vi "getBounds.vi"(0 "reference":refnum<class "StateDiagramGraph.lvclass">, 1 "graphics":refnum<class "Graphics.lvclass">, 5 "error in (no error)":errorcluster) -> (14 "reference out":refnum<class "StateDiagramGraph.lvclass">, 15 "bounds":T1 {"height" format="%.2f"; "width" format="%.2f"; "y" format="%.2f"; "x" format="%.2f"}, 19 "error out":errorcluster)   [LabVIEW 2014, in "StateDiagramGraph.lvclass"]
doc: "getBounds"
uses:
  <resource>/Framework/Providers/Open_GDS/UML/StateDiagramGraph_class/StateDiagramGraph.lvclass
  <resource>/Framework/Providers/Open_GDS/UML/Graphics_class/Graphics.lvclass
  <resource>/Framework/Providers/Open_GDS/UML/General/Rectangle/Rectangle Rectangle2D.ctl
  <resource>/Framework/Providers/Open_GDS/UML/StateDiagramGraph_class/private/ViPathShowOption.ctl
  <resource>/Framework/Providers/Open_GDS/UML/Graph_class/Graph.lvclass
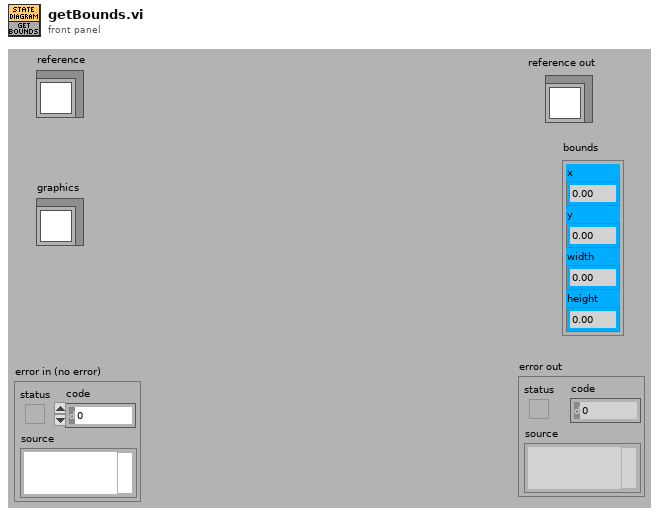
[diagram p1: front panel]
types:
  T1 = typedef "Rectangle Rectangle2D.ctl" = cluster{"x":dbl, "y":dbl, "width":dbl, "height":dbl}
  T2 = typedef "StateDiagramGraph.lvclass/ViPathShowOption.ctl" = enum16{"Don't Show", "Show Relative Path", "Show Absolute Path"}
  T3 = typedef "StateDiagramGraph.lvclass/ObjectAttributes.ctl" = cluster{"StateDiagramData":T4}
  T4 = typedef "StateDiagramGraph.lvclass/StateDiagramData.ctl" = cluster{"VI-Path":path, "ShowOption":T2}
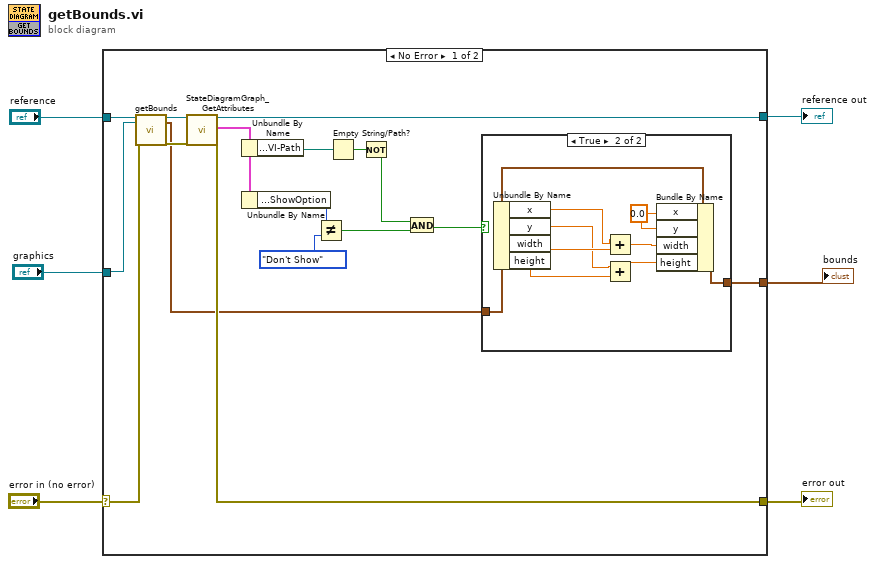
[diagram p0: block diagram]
diagram:
  n1 = case shown="No Error" "error in (no error)" {
    selector: "error in (no error)" -> [w10 w34]
    tunnel: "reference" -> [w13 w35]
    tunnel: [w22 w34] -> w4
    tunnel: [w23 w35] -> w3
    tunnel: "graphics" -> [w9 _]
    tunnel: [w21 _] -> w1
    frame No Error {
      n2 = call-parent "getBounds.vi"("reference"=w13, "graphics"=w9, "error in (no error)"=w10) -> ("reference out"=w12:refnum<class "StateDiagramGraph.lvclass">, "bounds"=w8:T1, "error out"=w11:errorcluster)  [unwired: 14 in]
      n3 = call <resource>:"StateDiagramGraph_GetAttributes.vi"("reference in"=w12, "error in (no error)"=w11) -> ("reference out"=w23:refnum<class "StateDiagramGraph.lvclass">, "Data"=w7:T3, "error out"=w22:errorcluster)  [unwired: 1 in, 14 out]
      n4 = Unbundle By Name(w7) -> ("StateDiagramData.VI-Path"=w17:path)
      n5 = Unbundle By Name(w7) -> ("StateDiagramData.ShowOption"=w20:T2)
      n6 = Not Equal?(x=w20, y=ViPathShowOption."Don't Show") -> (x != y?=w18:bool)
      n7 = Empty String/Path?(string/path=w17) -> (empty?=w16:bool)
      n8 = Not(x=w16) -> (.not. x?=w15:bool)
      n9 = And(x=w15, y=w18) -> (x .and. y?=w14:bool)
      n10 = case shown="True" w14 {
        tunnel: [w24 w33] -> w21
        tunnel: w8 -> [w24 w29]
        frame False {
        }
        frame True {
          w32 = 0.0 ("x")
          n11 = Unbundle By Name(w29) -> ("x"=w28:dbl, "y"=w26:dbl, "width"=w27:dbl, "height"=w25:dbl)
          n12 = Add(x=w28, y=w27) -> (x+y=w31:dbl)
          n13 = Add(x=w26, y=w25) -> (x+y=w30:dbl)
          n14 = Bundle By Name(cluster=w29, "x"=w32, "y"=w32, "width"=w31, "height"=w30) -> (w33:T1)
        }
      }
    }
    frame Error {
    }
  }
  "reference out" <- w3
  "error out" <- w4
  "bounds" <- w1
